vi "Setup Delay for Next State.vi"(8 "error in (no error)":errorcluster, 10 "Period":i32, 11 "Next State":string) -> (0 "error out":errorcluster)   [LabVIEW 2015, in "Tool Module.lvlib"]
uses:
  Tool Module.lvlib
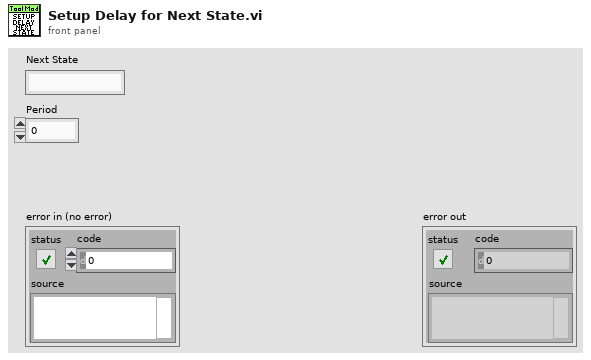
[diagram p1: front panel]
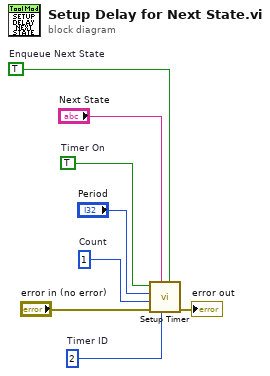
[diagram p0: block diagram]
diagram:
  w3 = 2  # Timer ID
  w4 = 1  # Count
  w5 = TRUE  # Timer On
  w8 = TRUE  # Enqueue Next State
  n1 = call "Setup Timer.vi"("Enqueue Next State"=w8, "Timer ID"=w3, "Next State"="Next State", "error in (no error)"="error in (no error)", "Count"=w4, "Period"="Period", "Timer On"=w5) -> ("error out"=→"error out":errorcluster)  [unwired: 4 in]
